vi "Read session.vi"(8 "error in (no error)":errorcluster, 11 "Scope PXI CFG in":refnum<class "Scope PXI CFG.lvclass">) -> (0 "error out":errorcluster, 2 "session":refnum<k15>, 3 "Scope PXI CFG out":refnum<class "Scope PXI CFG.lvclass">)   [LabVIEW 2023, in "HAL.lvlib" / "Scope PXI CFG.lvclass"]
uses:
  Scope PXI CFG.lvclass
  Scope PXI CFG.lvclass/Scope PXI CFG.ctl
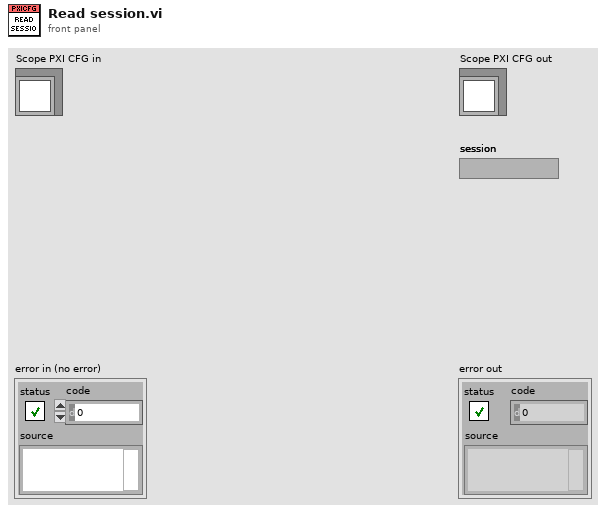
[diagram p1: front panel]
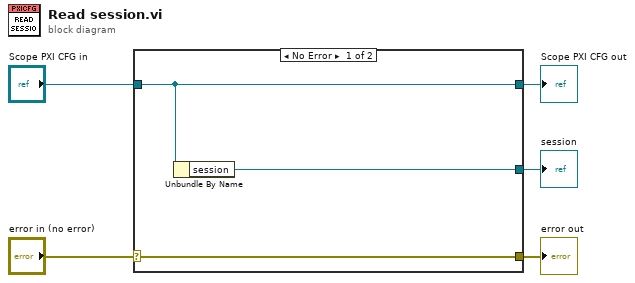
[diagram p0: block diagram]
diagram:
  n1 = case shown="No Error" "error in (no error)" {
    selector: "error in (no error)" -> [w8 w9]
    tunnel: [w8 w9] -> w4
    tunnel: [w7 w10] -> w2
    tunnel: "Scope PXI CFG in" -> [w7 w10]
    tunnel: [w6 _] -> w1
    frame No Error {
      n2 = Unbundle By Name(w7) -> ("session"=w6:refnum<k15>)
    }
    frame Error {
    }
  }
  "error out" <- w4
  "Scope PXI CFG out" <- w2
  "session" <- w1
